vi "两边沿间隔_有限.vi"() -> ()   [LabVIEW 2013]
uses:
  <userlib>/ArtDAQ/_SubVI/ArtDAQ_CreateCITwoEdgeSepChan.vi
  <userlib>/ArtDAQ/_SubVI/ArtDAQ_CfgImplicitTiming.vi
  <userlib>/ArtDAQ/_SubVI/ArtDAQ_Read Counter DBL NSamp.vi
panel:
  in  "第二个边沿":i32(ring)=10280 items=["上升"=10280, "下降"=10171]
  in  "第一个边沿":i32(ring)=10280 items=["上升"=10280, "下降"=10171]
  in  "每通道点数":i32=100
  in  "Stop":bool
  out "数据":dbl[](array[numeric])
  in  "计数器":string="Dev1/ctr0"
  in  "最小值":dbl=1e-06 format="%0.6f"
  in  "最大值":dbl=10.0 format="%0.6f"
  out "错误输出":errorcluster
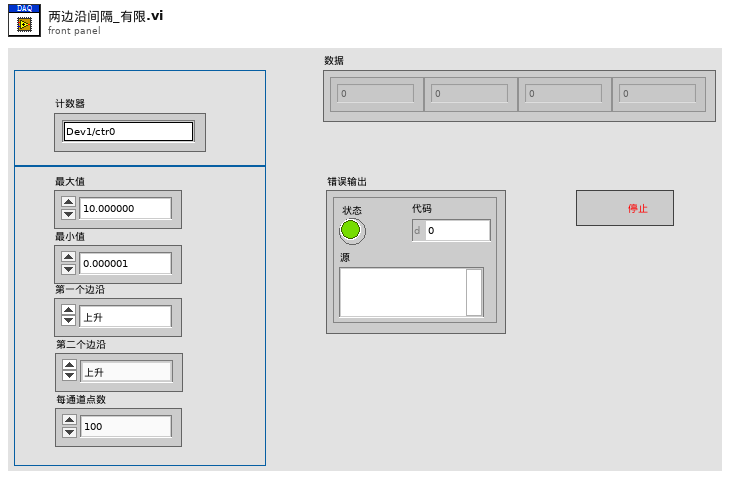
[diagram p1: front panel]
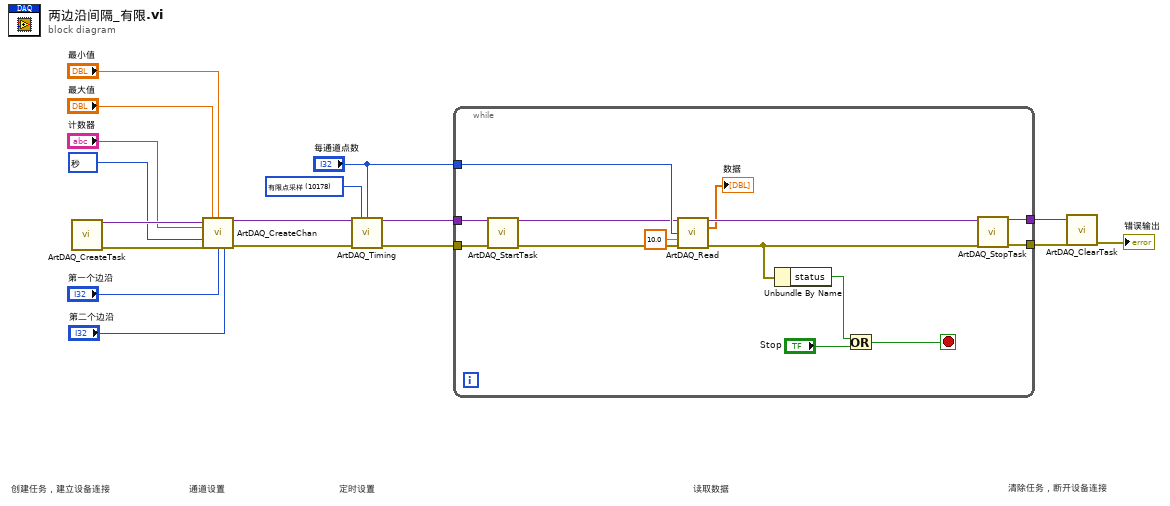
[diagram p0: block diagram]
diagram:
  w3 = 10364 items=["秒"=10364, "时钟滴答"=10304, "来自自定义换算"=10065] ("Units")
  w7 = 10178 items=["有限点采样"=10178, "连续采样"=10123] ("SampleMode")
  # "清除任务，断开设备连接"
  # "读取数据"
  # "定时设置"
  # "通道设置"
  # "创建任务，建立设备连接"
  n1 = call <userlib>:"ArtDAQ_CreateTask.vi"() -> ("任务句柄"=w17:variant, "错误输出"=w16:errorcluster)  [unwired: 14 in]
  n2 = call-poly <userlib>:"ArtDAQ_CreateChan.vi"("任务句柄"=w17, "最大值"="最大值", "最小值"="最小值", "计数器"="计数器", "单位"=w3, "错误输入"=w16, "第一个边沿"="第一个边沿", "第二个边沿"="第二个边沿") -> ("任务句柄"=w9:variant, "错误输出"=w8:errorcluster)  [unwired: 6 in]
  n3 = call-poly <userlib>:"ArtDAQ_Timing.vi"("任务句柄"=w9, "采样模式"=w7, "每通道采样数"="每通道点数", "错误输入"=w8) -> ("任务句柄"=w5:variant, "错误输出"=w4:errorcluster)  [unwired: 10 in]
  n4 = while {
    tunnel: [w30] -> w14
    tunnel: [w28] -> w13
    tunnel: "每通道点数" -> [w27]
    tunnel: w5 -> [w26]
    tunnel: w4 -> [w25]
    stop <- w18 stop-if-true
    n5 = call <userlib>:"ArtDAQ_StartTask.vi"("任务句柄"=w26, "错误输入"=w25) -> ("任务句柄"=w20:variant, "错误输出"=w19:errorcluster)  [unwired: 12 in]
    n6 = call-poly <userlib>:"ArtDAQ_Read.vi"("任务句柄"=w20, "每通道采样数"=w27, "超时s"=10.0 ("Timeout"), "错误输入"=w19) -> ("任务句柄"=w31:variant, "数据"=→"数据":dbl[], "错误输出"=w29:errorcluster)  [unwired: 8 in, 1 out]
    n7 = Unbundle By Name(w29) -> ("status"=w22:bool)
    n8 = Or(x=w22, y="Stop") -> (x .or. y?=w18:bool)
    n9 = call <userlib>:"ArtDAQ_StopTask.vi"("任务句柄"=w31, "错误输入"=w29) -> ("任务句柄"=w30:variant, "错误输出"=w28:errorcluster)  [unwired: 12 in]
  }
  n10 = call <userlib>:"ArtDAQ_ClearTask.vi"("任务句柄"=w14, "错误输入"=w13) -> ("错误输出"=→"错误输出":errorcluster)  [unwired: 13 in]
